vi "Home.vi"(8 "error in (no error)":errorcluster, 11 "DemoStepMotor in":refnum<class "DemoStepMotor.lvclass">) -> (0 "error out":errorcluster, 3 "DemoStepMotor out":refnum<class "DemoStepMotor.lvclass">)   [LabVIEW 2020, in "DemoStepMotor.lvlib" / "DemoStepMotor.lvclass"]
uses:
  DemoStepMotor.lvclass
  Hardware Abstraction Layer/Component/Stage/Stage/Stage.lvclass
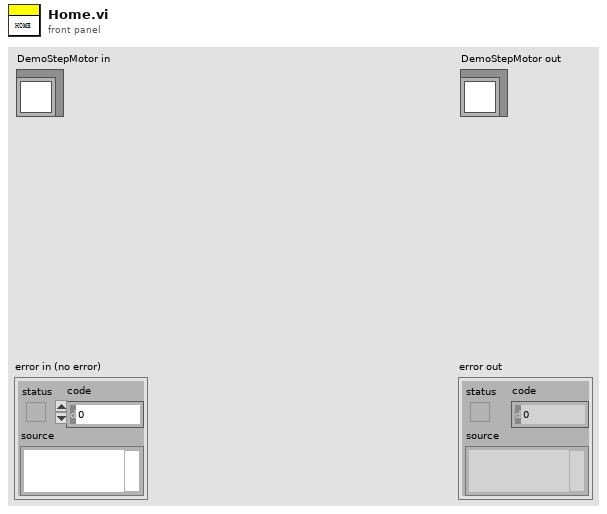
[diagram p1: front panel]
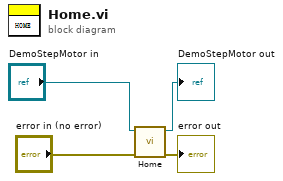
[diagram p0: block diagram]
diagram:
  n1 = call-parent "Home.vi"("error in (no error)"="error in (no error)", "Stage in"="DemoStepMotor in") -> ("error out"=→"error out":errorcluster, "Stage out"=→"DemoStepMotor out":refnum<class "DemoStepMotor.lvclass">)  [unwired: 8 in]
